vi "Write File with flush (string).vi"(4 "convert eol? (no:F)":bool, 5 "string":string, 6 "Flush interval (s)":dbl=60.0 format="%.2f", 7 "error in (no error)":errorcluster, 8 "pos offset (bytes:0)":i32, 9 "pos mode (rel. to end:1)":enum16{"start", "end", "current"}(ring)=enum."end", 10 "refnum":refnum<file>) -> (0 "error out":errorcluster, 1 "mark after write (bytes)":i32, 3 "dup refnum":refnum<file>)   [LabVIEW 2015]
doc: "Writes a string of characters to a byte stream file at the specified location; the default location is at the end of file. The VI does incoming and internal error checking and does not write if an incoming error occurs.\n\nrefnum is the reference number of the open file.\n\npos mode specifies where the write begins relative to pos offset:\n\n 0: at the beginning of the file plus pos offset.\n\n 1: at the end of the file plus pos offset. This is the default value.\n\n 2: at the current file mark plus pos offset.\n\npos offset specifies in characters how far from the location specified by pos mode that the operation begins. The default value is 0.\n\ncharacter string is the data the VI writes to the file.\n\nconvert eol Set TRUE to convert the LabVIEW end of line marker to the platform-specific marker. Set FALSE (default value) to do nothing.\n\nerror in is a cluster of three elements (error?, code, and source) that describe the upstream error state, that is, the existance of any error preceeding the execution of the VI. The VI executes normally only if no incoming error exists; otherwise it merely passes the error in value to error out. error? is TRUE if an error occurred; the default value is FALSE. code is the error code; the default value is 0. source is in most cases the name of the VI or function that produced the error; the default value is an empty string.\n\ndup refnum is a flow-though parameter with the same value as refnum.\n\nmark after write is the location of the character following the last character written.\n\nerror out is a cluster of three elements (error?, code, and source) that describe the error state following the execution of the VI. If an incoming error does not exist, the VI executes normally and error out describes the VI's error state; if an incoming error exists, error out equals error in."
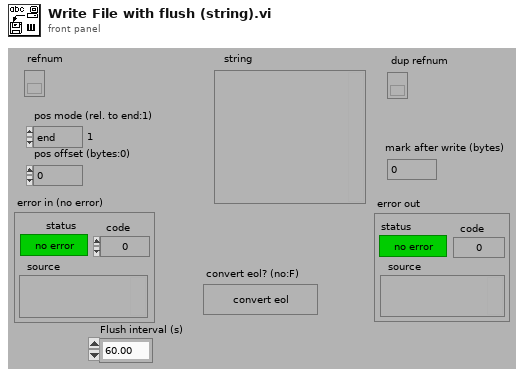
[diagram p1: front panel]
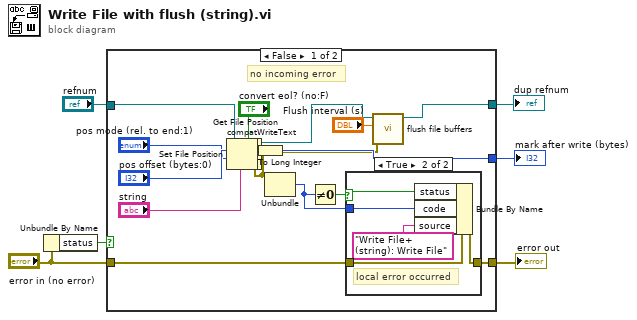
[diagram p0: block diagram]
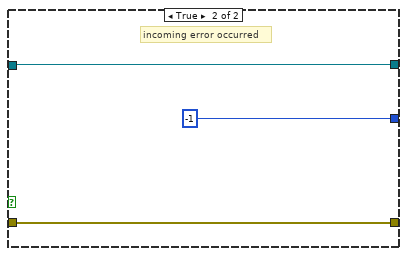
[diagram p3: hidden frame]
diagram:
  n1 = Unbundle By Name("error in (no error)") -> ("status"=w6:bool)
  n2 = case shown="False" w6 {
    tunnel: [w20 w33] -> w5
    tunnel: [w23 -1] -> w4
    tunnel: [w14 w32] -> w3
    tunnel: "refnum" -> [w22 w32]
    tunnel: "error in (no error)" -> [w19 w33]
    frame False {
      # "no incoming error"
      n3 = Set File Position(offset (in bytes) (0)="pos offset (bytes:0)", refnum=w22, from (0:start)="pos mode (rel. to end:1)") -> (refnum out=w11:refnum<file>, error out=w10:errorcluster)  [unwired: 1 in]
      n4 = call <vilib>:"compatWriteText.vi"("convert eol (F)"="convert eol? (no:F)", "data"="string", "error in"=w10, "refnum"=w11) -> ("error out"=w8:errorcluster, "dup refnum"=w9:refnum<file>)  [unwired: 6 in]
      n5 = Get File Position(4:w8, 7:w9) -> (0:w13:errorcluster, 2:w7:i64, 3:w15:refnum<file>)
      n6 = To Long Integer(number=w7) -> (32bit integer=w23:i32)
      n7 = Unbundle(w13) -> ("code"=w17:i32)  [unwired: 2 out]
      n8 = Not Equal To 0?(x=w17) -> (x != 0?=w18:bool)
      n9 = case shown="True" w18 {
        selector: w18 -> [_ w27]
        tunnel: w17 -> [_ w30]
        tunnel: [w26 w28] -> w20
        tunnel: w19 -> [w26 w29]
        frame False {
          # "no local error"
        }
        frame True {
          # "local error occurred"
          n10 = Bundle By Name(cluster=w29, "status"=w27, "code"=w30, "source"="Write File+ (string): Write File") -> (w28:errorcluster)
        }
      }
      n11 = call "flush file buffers.vi"("error in"=w13, "Flush interval (s)"="Flush interval (s)", "refnum"=w15) -> ("dup refnum"=w14:refnum<file>)  [unwired: 7 in, 1 out]
    }
    frame True {
      # "incoming error occurred"
    }
  }
  "error out" <- w5
  "mark after write (bytes)" <- w4
  "dup refnum" <- w3
